vi "SetTimeConstant.vi"(8 "error in":errorcluster, 10 "Time Const":T1(ring), 11 "Port":refnum<visa-resource-name>) -> (0 "error out":errorcluster, 3 "Port out":refnum<visa-resource-name>)   [LabVIEW 2018]
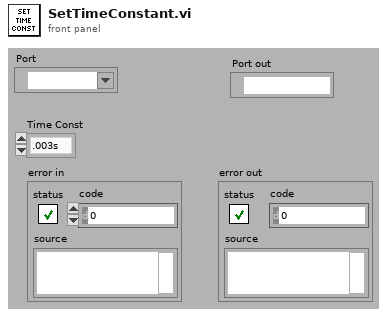
[diagram p1: front panel]
types:
  T1 = enum16{".003s", ".010s", ".030s", ".100s", ".300s", "1.00s", "3.00s", "10.0s", "30.0s", "100s"}
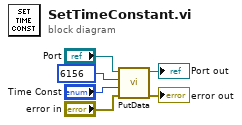
[diagram p0: block diagram]
diagram:
  n1 = call "PutData.vi"("error in"="error in", "Value"="Time Const", "Location"=u32 6156, "Port"="Port") -> ("error out"=→"error out":errorcluster, "Port out"=→"Port out":refnum<visa-resource-name>)  [unwired: 6 in]
